vi "E8267D GetFrequency.vi"(0 "VISA Rsrc":refnum<visa-resource-name>="GPIB0::12::INSTR", 5 "FUnits":u16(ring) caption="Units" items=["Hz", "MHz", "GHz"], 11 "error in (no error)":errorcluster) -> (4 "VISA Rsrc Out":refnum<visa-resource-name>="GPIB0::12::INSTR", 6 "Frequency (Hz)":dbl, 8 "Frequency (Units)":dbl, 15 "error out":errorcluster)   [LabVIEW 2019]
doc: "Ce VI écrit les paramètres de la zone de contrôle spécifiée dans le contrôlleur"
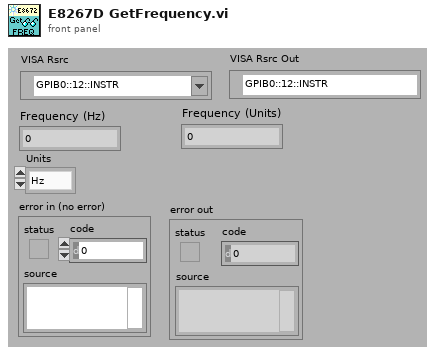
[diagram p1: front panel]
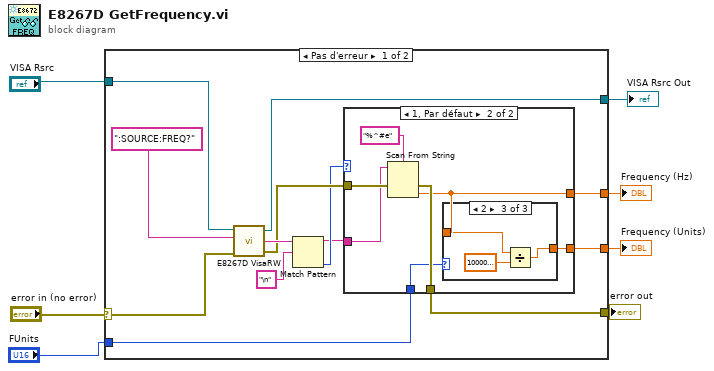
[diagram p0: block diagram]
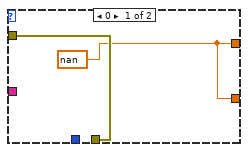
[diagram p2: hidden frame]
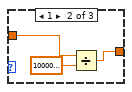
[diagram p4: hidden frame]
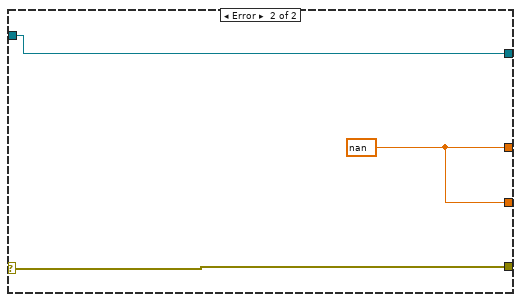
[diagram p5: hidden frame]
diagram:
  n1 = case shown="Pas d'erreur" "error in (no error)" {
    selector: "error in (no error)" -> [w20 w39]
    tunnel: "VISA Rsrc" -> [w19 w38]
    tunnel: [w14 w39] -> w6
    tunnel: [w17 w38] -> w4
    tunnel: [w13 w37] -> w3
    tunnel: [w9 w37] -> w2
    tunnel: "FUnits" -> [w8 _]
    frame No Error {
      n2 = call <userlib>:"E8267D VisaRW.vi"("error in (no error)"=w20, "ChaineCom"=":SOURCE:FREQ?", "VISA Rsrc"=w19) -> ("error out"=w15:errorcluster, "ChaineRep"=w16:string, "VISA Rsrc Out"=w17:refnum<visa-resource-name>)  [unwired: 4 in, 1 out]
      n3 = Match Pattern(string=w16, regular expression="\n" ("expression régulière")) -> (before substring=w10:string, offset past match=w11:i32)  [unwired: 1 in, 2 out]
      n4 = case shown="1, Par défaut" w11 {
        tunnel: w15 -> [w22 w29]
        tunnel: [w22 w28] -> w14
        tunnel: [w21 w23] -> w13
        tunnel: w10 -> [_ w26]
        tunnel: [w21 w24] -> w9
        tunnel: w8 -> [_ w25]
        frame 0 {
          w21 = nan
        }
        frame 1, Default {
          n5 = Scan From String(format string="%^#e" ("chaîne de format"), input string=w26, error in=w29) -> (error out=w28:errorcluster, output 1=w23:dbl)  [unwired: 2 in, 2 out]
          n6 = case shown="2" w25 {
            tunnel: [w30 w33 w36] -> w24
            tunnel: w23 -> [w30 w32 w35]
            frame 0, Default {
            }
            frame 1 {
              n7 = Divide(x=w32, y=1000000.0) -> (x/y=w33:dbl)
            }
            frame 2 {
              n8 = Divide(x=w35, y=1000000000.0) -> (x/y=w36:dbl)
            }
          }
        }
      }
    }
    frame Error {
      w37 = nan
    }
  }
  "error out" <- w6
  "Frequency (Hz)" <- w3
  "VISA Rsrc Out" <- w4
  "Frequency (Units)" <- w2
